vi "instantiateTwoTcpServer.vi"(8 "error in (no error)":errorcluster, 11 "FactoryTcpServer in":refnum<class "FactoryTcpServer.lvclass">) -> (0 "error out":errorcluster, 1 "FactoryTcpServer out":refnum<class "FactoryTcpServer.lvclass">, 2 "TcpServer 2 out":refnum<class "TcpServer.lvclass">, 3 "TcpServer 1 out":refnum<class "TcpServer.lvclass">)   [LabVIEW 2018]
doc: "This create two instances of TcpServer"
uses:
  src/TcpServer/TcpServer.lvclass
  src/FactoryTcpServer/FactoryTcpServer.lvclass
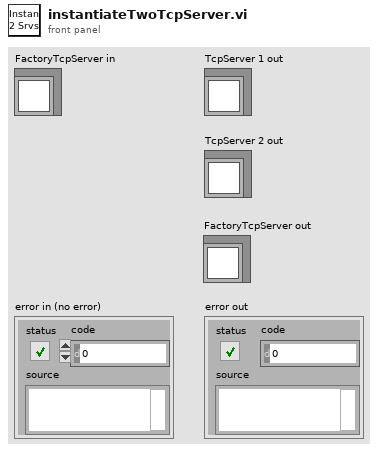
[diagram p1: front panel]
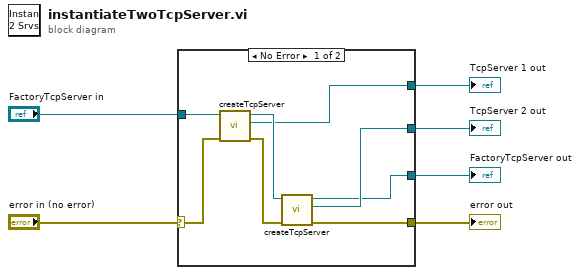
[diagram p0: block diagram]
diagram:
  n1 = case shown="No Error" "error in (no error)" {
    selector: "error in (no error)" -> [w12 w15]
    tunnel: [w14 w15] -> w6
    tunnel: "FactoryTcpServer in" -> [w10 _]
    tunnel: [w9 _] -> w3
    tunnel: [w8 _] -> w2
    tunnel: [w7 _] -> w1
    frame No Error {
      n2 = call "createTcpServer.vi"("error in (no error)"=w12, "FactoryTcpServer in"=w10) -> ("error out"=w13:errorcluster, "TcpServer out"=w9:refnum<class "TcpServer.lvclass">, "FactoryTcpServer out"=w11:refnum<class "FactoryTcpServer.lvclass">)  [unwired: 7 in]
      n3 = call "createTcpServer.vi"("error in (no error)"=w13, "FactoryTcpServer in"=w11) -> ("error out"=w14:errorcluster, "TcpServer out"=w8:refnum<class "TcpServer.lvclass">, "FactoryTcpServer out"=w7:refnum<class "FactoryTcpServer.lvclass">)  [unwired: 7 in]
    }
    frame Error {
    }
  }
  "error out" <- w6
  "TcpServer 1 out" <- w3
  "TcpServer 2 out" <- w2
  "FactoryTcpServer out" <- w1
